vi "Get Boolean Package Attribute Value.vi"(8 "error in (no error)":errorcluster, 10 "package attribute name":string, 11 "package attributes CLI string":string) -> (0 "error out":errorcluster, 3 "package attribute value":bool)   [LabVIEW 2014, in "NIPM_API.lvlib"]
uses:
  NIPM_API.lvlib
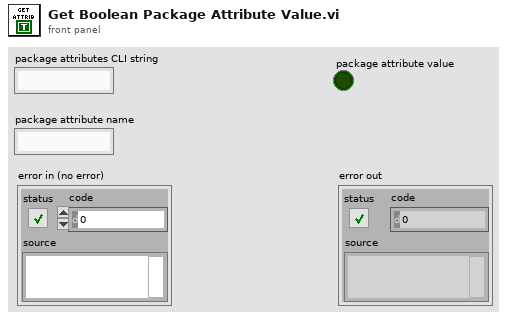
[diagram p1: front panel]
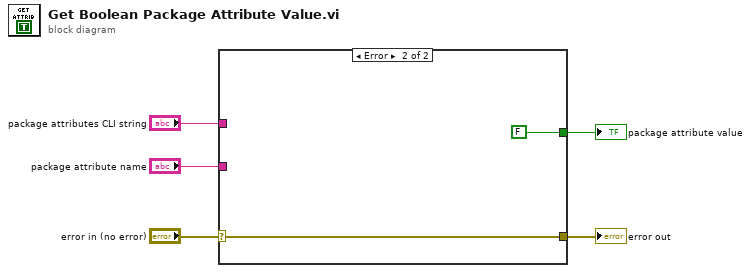
[diagram p0: block diagram]
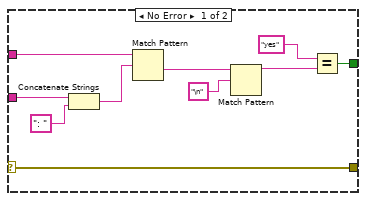
[diagram p2: hidden frame]
diagram:
  n1 = case shown="Error" "error in (no error)" {
    selector: "error in (no error)" -> [w6 w17]
    tunnel: "package attribute name" -> [w15 _]
    tunnel: "package attributes CLI string" -> [w14 _]
    tunnel: [w13 FALSE] -> w3
    tunnel: [w6 w17] -> w1
    frame No Error {
      n2 = Concatenate Strings(w15, ": " ("string")) -> (w9:string)
      n3 = Match Pattern(string=w14, regular expression=w9) -> (after substring=w10:string)  [unwired: 1 in, 3 out]
      n4 = Match Pattern(string=w10, regular expression="\n") -> (before substring=w12:string)  [unwired: 1 in, 3 out]
      n5 = Equal?(x="yes", y=w12) -> (x = y?=w13:bool)
    }
    frame Error {
    }
  }
  "package attribute value" <- w3
  "error out" <- w1
